vi "ML.vi"(8 "error in (no error)":errorcluster, 11 "Agilis in":T1) -> (0 "error out":errorcluster, 3 "Agilis out":T1)   [LabVIEW 2016, in "Drivers.lvlib" / "Agilis.lvlib"]
doc: "Sets the controller to local mode. In local mode the pushbuttons on the controller are enabled and all commands that configure or operate the controller are disabled."
uses:
  Agilis.lvlib
  AgilisCmdLib Refnum.ctl
  Z:/TraceGrabber/Drivers/Agilis/AgilisCmdLib.dll
  AgilisCmdLib.dll
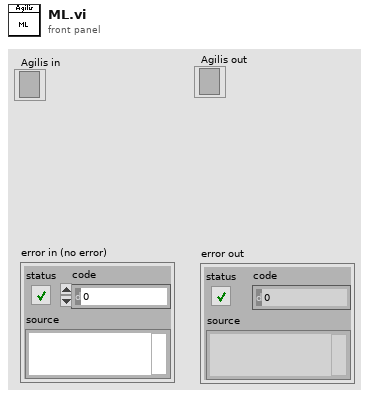
[diagram p1: front panel]
types:
  T1 = typedef "Drivers.lvlib/Agilis.lvlib/AgilisCmdLib Refnum.ctl" = refnum<k24>
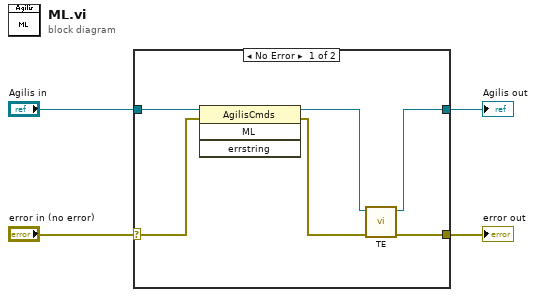
[diagram p0: block diagram]
diagram:
  n1 = case shown="No Error" "error in (no error)" {
    selector: "error in (no error)" -> [w9 w12]
    tunnel: "Agilis in" -> [w10 w11]
    tunnel: [w5 w11] -> w2
    tunnel: [w8 w12] -> w1
    frame No Error {
      n2 = invoke class="AgilisCmds" method="ML"(reference=w10, error in=w9) -> (reference out=w6:T1, error out=w7:errorcluster)  [unwired: 2 in, 2 out]
      n3 = call "TE.vi"("error in (no error)"=w7, "Agilis in"=w6) -> ("error out"=w8:errorcluster, "Agilis out"=w5:T1)  [unwired: 8 in]
    }
    frame Error {
    }
  }
  "Agilis out" <- w2
  "error out" <- w1
